vi "~Selectors.vi"() -> ()   [LabVIEW 2017]
uses:
  Classes/Sequence/SequenceSubvis/TestStep.ctl
  Classes/Sequence/SequenceSubvis/RF Direction.ctl
  Classes/Sequence/SequenceSubvis/PolarizationSelect.ctl
panel:
  in  "module 8":T1
  in  "module 7":T1
  in  "module 6":T1
  in  "module 5":T1
  in  "module 4":T1
  in  "module 3":T1
  in  "module 2":T1
  in  "module":T2
  out "Test Sequence":T3[](array[typedef])
  in  "Rx":bool
  in  "Tx":bool
  in  "Horizontal":T6
  in  "Vertical":T6
  in  "Selector":bool[][](array[boolean])=[[TRUE, FALSE, FALSE, FALSE, FALSE, FALSE, FALSE, FALSE], [FALSE, FALSE, FALSE, FALSE, FALSE, FALSE, FALSE, FALSE], [TRUE, FALSE, FALSE, FALSE, FALSE, FALSE, FALSE, FALSE], [FALSE, FALSE, FALSE, FALSE, FALSE, FALSE, FALSE, FALSE]] caption="0     1     2     3     4    5     6     7"
  # "Module #"
  # "Tx Vertical"
  # "Tx Horizontal"
  # "Rx Vertical"
  # "Rx Horizontal"
  # "Tx Vertical"
  # "Tx Horizontal"
  # "Rx Vertical"
  # "Rx Horizontal"
  # "Module 0"
  # "Module 1"
  # "Module 2"
  # "Module 3"
  # "Module 4"
  # "Module 5"
  # "Module 6"
  # "Module 7"
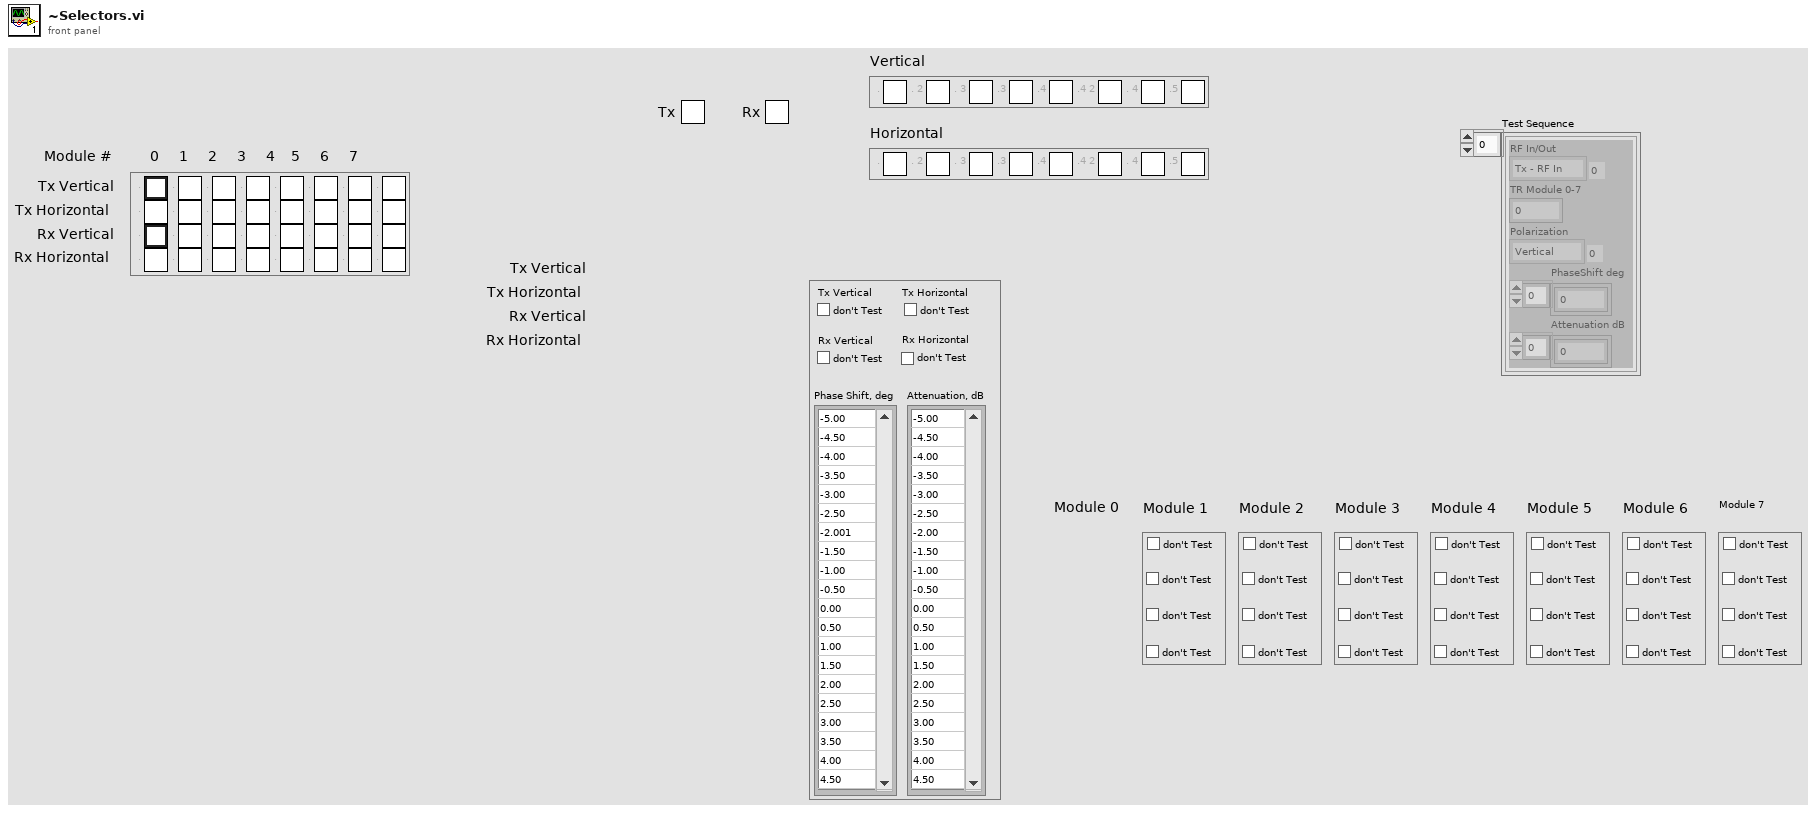
[diagram p1: front panel]
types:
  T1 = cluster{"Tx Vertical":bool, "Tx Horizontal":bool, "Rx Vertical":bool, "Tx Horizontal 2":bool}
  T2 = cluster{"Tx Vertical":bool, "Tx Horizontal":bool, "Rx Vertical":bool, "Rx Horizontal":bool, "Attenuation, dB":i32[], "Phase Shift, deg":i32[]}
  T3 = typedef "TestStep.ctl" = cluster{"RF In/Out":T4, "TR Module 0-7":i32, "Polarization":T5, "PhaseShift deg":dbl[], "Attenuation dB":dbl[]}
  T4 = typedef "RF Direction.ctl" = enum16{"Tx - RF In", "Rx - RF Out"}
  T5 = typedef "PolarizationSelect.ctl" = enum16{"Vertical", "Horizontal"}
  T6 = cluster{" .":bool, " . 2":bool, " . 3":bool, " .3":bool, " .4":bool, " .4 2":bool, " . 4":bool, " .5":bool}
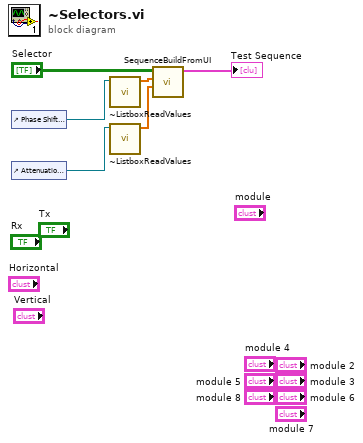
[diagram p0: block diagram]
diagram:
  n1 = control-ref of="Phase Shift, deg"() -> (w6:refnum<vi>)
  n2 = control-ref of="Attenuation, dB"() -> (w5:refnum<vi>)
  n3 = call "~ListboxReadValues.vi"("Listbox Ref"=w6) -> ("Selected Values"=w4:dbl[])  [unwired: 10 in]
  n4 = call "~ListboxReadValues.vi"("Listbox Ref"=w5) -> ("Selected Values"=w3:dbl[])  [unwired: 10 in]
  n5 = call "SequenceBuildFromUI.vi"("Attenuations, dB"=w3, "Phase Shifts, deg"=w4, "2D Selector"="Selector") -> ("Test Sequence"=→"Test Sequence":T3[])  [unwired: 8 in]
